vi "TurnForTime.vi"() -> ()   [LabVIEW 2018]
uses:
  Framework/Robot Global Data.vi
panel:
  in  "NoWait":bool
  in  "Time":dbl
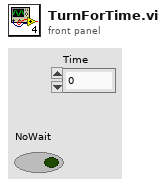
[diagram p1: front panel]
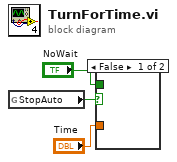
[diagram p0: block diagram]
diagram:
  n1 = global read "Robot Global Data.vi" "StopAuto"() -> (w1:bool)
  n2 = case shown="False" w1 {
    tunnel: "Time" -> [_ _]
    tunnel: "NoWait" -> [_ _]
    frame False {
    }
    frame True {
    }
  }
